vi "Build Dashboard Data.vi"(11 "Dashboard Enables":T3={"Analog Module 1"=[TRUE, TRUE, TRUE, TRUE, TRUE, TRUE, TRUE, TRUE], "Analog Module 2"=[FALSE, FALSE, FALSE, FALSE, FALSE, FALSE, FALSE, FALSE], "Digital Module 1"=TRUE, "Digital Module 2"=FALSE, "Solenoid Module"=FALSE, "Turret Gyro"=TRUE, "Robot Gyro"=TRUE, "Left Encoder"=TRUE, "Launcher Rate"=TRUE, "Right Encoder"=TRUE, "Drive Distance"=TRUE, "Selected Target"=TRUE, "Target Info"=TRUE, "Target Distance"=TRUE, "Bounding Box"=TRUE}) -> ()   [LabVIEW 2012]
doc: "This VI builds data and sends it back to the dashboard PC program. By default it sends back the raw values for the first analog, digital, and solenoid module. Modify it to send back the data you want to view. Consider adding higher level data to the Dashboard Datatype.ctl and to this VI. Then update the Dashboard to display the data however you like.\n\nThis software is licensed. Open the labview\\readme\\WPI Robotics Library Open Source License.txt file for more information."
uses:
  Dashboard Datatype.ctl
  <vilib>/Rock Robotics/WPI/DriverStation/WPI_DriverStationDigitalData.ctl
  <vilib>/Rock Robotics/SystemInterfaces/System/FPGA_SystemGet.vi
  Robot Global Data.vi
panel:
  out "Dashboard Data":T1
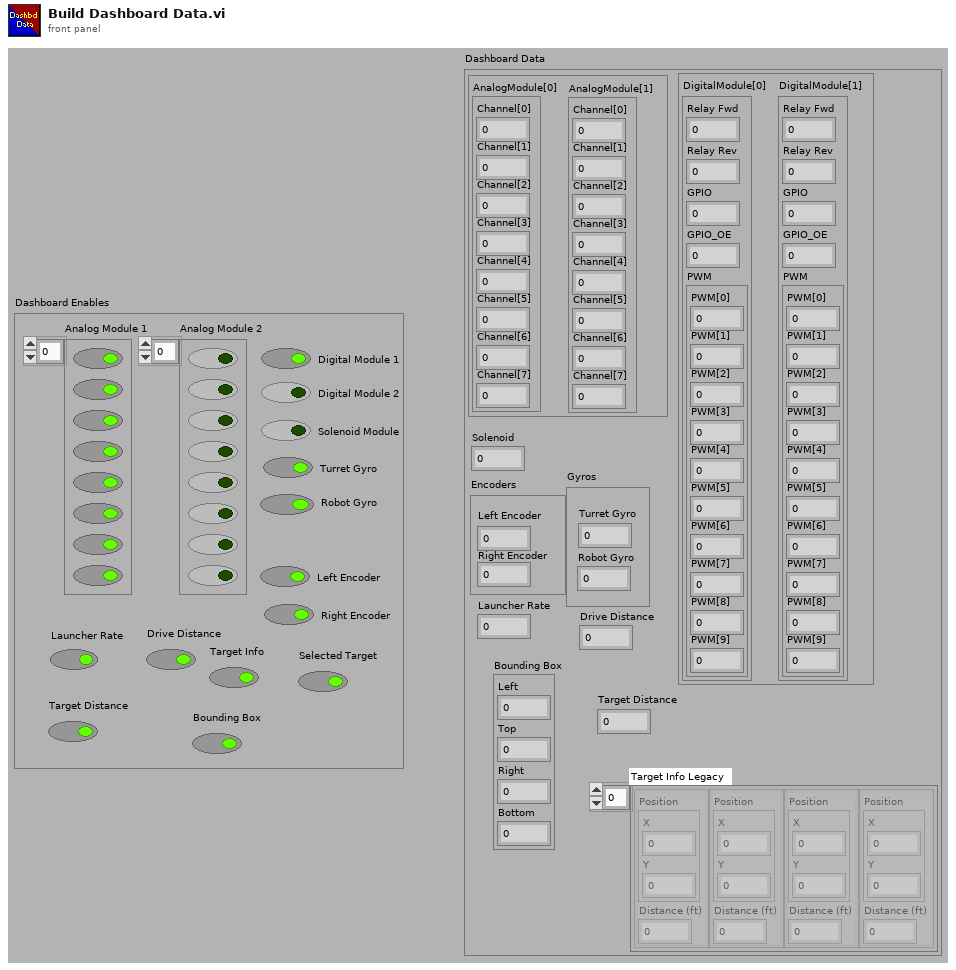
[diagram p1: front panel]
types:
  T1 = typedef "Dashboard Datatype.ctl" = cluster{cluster{"AnalogModule[0]":cluster{"Channel[0]":sgl, "Channel[1]":sgl, "Channel[2]":sgl, "Channel[3]":sgl, "Channel[4]":sgl, "Channel[5]":sgl, "Channel[6]":sgl, "Channel[7]":sgl}, "AnalogModule[1]":cluster{"Channel[0]":sgl, "Channel[1]":sgl, "Channel[2]":sgl, "Channel[3]":sgl, "Channel[4]":sgl, "Channel[5]":sgl, "Channel[6]":sgl, "Channel[7]":sgl}}, cluster{"DigitalModule[0]":T2, "DigitalModule[1]":T2}, "Solenoid":u8, "Launcher Rate":dbl, "Gyros":cluster{"Turret Gyro":dbl, "Robot Gyro":dbl}, "Encoders":cluster{"Left Encoder":dbl, "Right Encoder":dbl}, "Drive Distance":dbl, "Bounding Box":cluster{"Left":dbl, "Top":dbl, "Right":dbl, "Bottom":dbl}, "Target Distance":dbl, "Target Info Legacy":cluster{"Position":cluster{"X":dbl, "Y":dbl}, "Distance (ft)":dbl}[]}
  T2 = typedef "WPI_DriverStationDigitalData.ctl" = cluster{"Relay Fwd":u8, "Relay Rev":u8, "GPIO":u16, "GPIO_OE":u16, "PWM":cluster{"PWM[0]":u8, "PWM[1]":u8, "PWM[2]":u8, "PWM[3]":u8, "PWM[4]":u8, "PWM[5]":u8, "PWM[6]":u8, "PWM[7]":u8, "PWM[8]":u8, "PWM[9]":u8}}
  T3 = cluster{"Analog Module 1":bool[], "Analog Module 2":bool[], "Digital Module 1":bool, "Digital Module 2":bool, "Solenoid Module":bool, "Turret Gyro":bool, "Robot Gyro":bool, "Left Encoder":bool, "Launcher Rate":bool, "Right Encoder":bool, "Drive Distance":bool, "Selected Target":bool, "Target Info":bool, "Target Distance":bool, "Bounding Box":bool}
  T4 = cluster{"AnalogModule[0]":cluster{"Channel[0]":sgl, "Channel[1]":sgl, "Channel[2]":sgl, "Channel[3]":sgl, "Channel[4]":sgl, "Channel[5]":sgl, "Channel[6]":sgl, "Channel[7]":sgl}, "AnalogModule[1]":cluster{"Channel[0]":sgl, "Channel[1]":sgl, "Channel[2]":sgl, "Channel[3]":sgl, "Channel[4]":sgl, "Channel[5]":sgl, "Channel[6]":sgl, "Channel[7]":sgl}}
  T5 = cluster{"Channel[0]":sgl, "Channel[1]":sgl, "Channel[2]":sgl, "Channel[3]":sgl, "Channel[4]":sgl, "Channel[5]":sgl, "Channel[6]":sgl, "Channel[7]":sgl}[]
  T6 = cluster{"Channel[0]":sgl, "Channel[1]":sgl, "Channel[2]":sgl, "Channel[3]":sgl, "Channel[4]":sgl, "Channel[5]":sgl, "Channel[6]":sgl, "Channel[7]":sgl}
  T7 = cluster{"AnalogModule[0][0]":sgl, "AnalogModule[0][1]":sgl, "AnalogModule[0][2]":sgl, "AnalogModule[0][3]":sgl, "AnalogModule[0][4]":sgl, "AnalogModule[0][5]":sgl, "AnalogModule[0][6]":sgl, "AnalogModule[0][7]":sgl}
  T8 = cluster{"[0]":cluster{"Channel[0]":sgl, "Channel[1]":sgl, "Channel[2]":sgl, "Channel[3]":sgl, "Channel[4]":sgl, "Channel[5]":sgl, "Channel[6]":sgl, "Channel[7]":sgl}, "[1]":cluster{"Channel[0]":sgl, "Channel[1]":sgl, "Channel[2]":sgl, "Channel[3]":sgl, "Channel[4]":sgl, "Channel[5]":sgl, "Channel[6]":sgl, "Channel[7]":sgl}}
  T9 = cluster{"DigitalModule[0]":T2, "DigitalModule[1]":T2}
  T10 = typedef "FPGA_DIODevRef.ctl" = cluster{"DevStatus":errorcluster, "Module":T11}
  T11 = typedef "FPGA_TypedefDigitalModule.ctl" = enum16{"Digital Module 1", "Digital Module 2"}
  T12 = cluster{"[0]":u8, "[1]":u8, "[2]":u8, "[3]":u8, "[4]":u8, "[5]":u8, "[6]":u8, "[7]":u8, "[8]":u8, "[9]":u8}
  T13 = cluster{"Left":dbl, "Top":dbl, "Right":dbl, "Bottom":dbl}
  T14 = typedef "FPGA_SolenoidDevRef.ctl" = cluster{"DevStatus":errorcluster, "Module":T15}
  T15 = typedef "FPGA_TypedefSolenoidModule.ctl" = enum16{"Solenoid Module 1", "Solenoid Module 2"}
  T16 = cluster{"Position":cluster{"X":dbl, "Y":dbl}, "Distance (ft)":dbl}[]
  T17 = typedef "WPI_GyroDevRef.ctl" = cluster{"DevStatus":errorcluster, "Analog Module":T18, "Analog Channel":T19, "Offset":dbl, "Gain (VoltsPerDegree/Second)":dbl}
  T18 = typedef "FPGA_TypedefAnalogModule.ctl" = enum16{"Analog Module 1", "Analog Module 2"}
  T19 = typedef "FPGA_AIChannel.ctl" = enum8{"AI 1", "AI 2", "AI 3", "AI 4", "AI 5", "AI 6", "AI 7", "AI 8", "Invalid"}
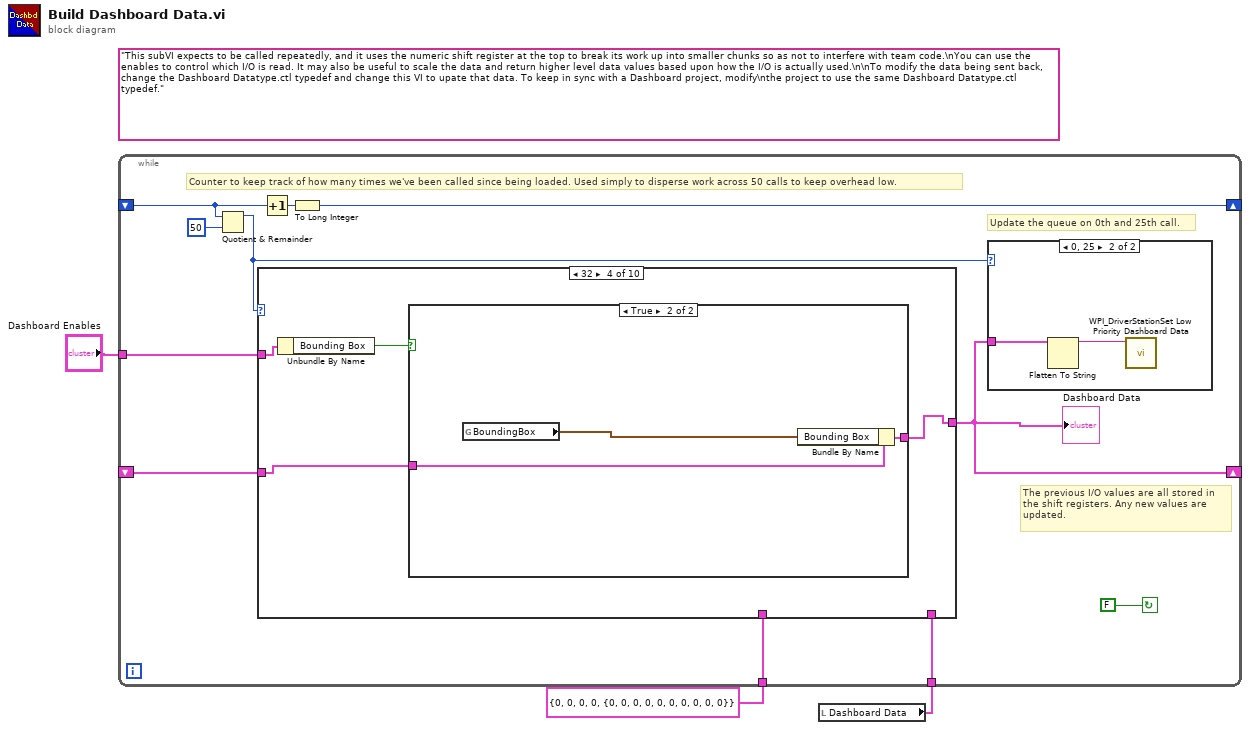
[diagram p0: block diagram]
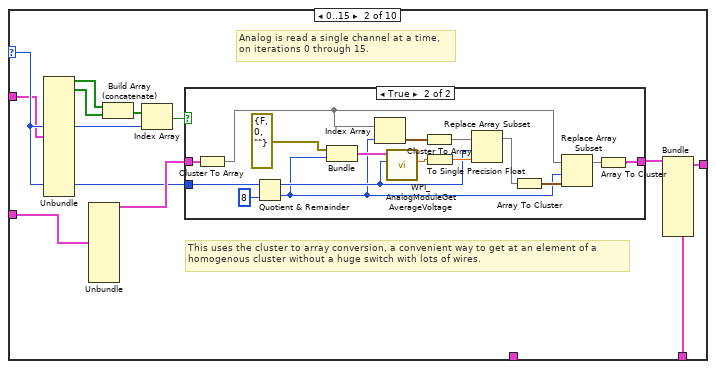
[diagram p4: hidden frame]
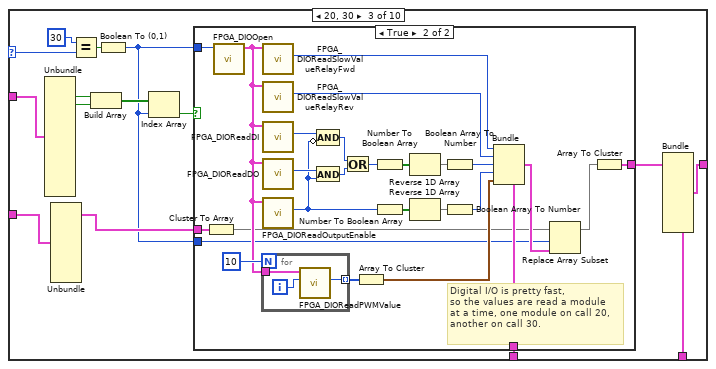
[diagram p6: hidden frame]
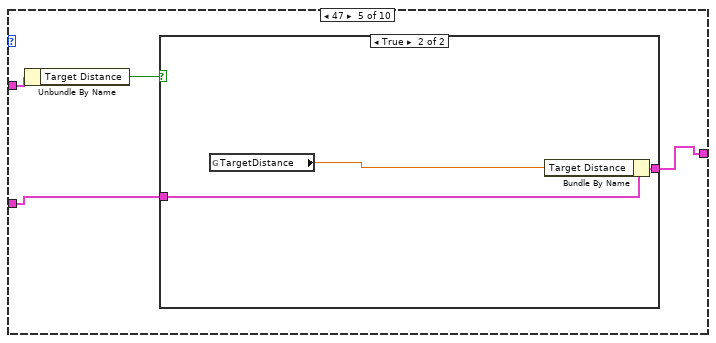
[diagram p9: hidden frame]
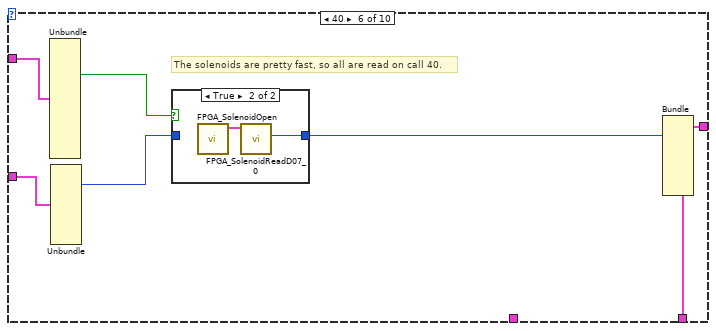
[diagram p11: hidden frame]
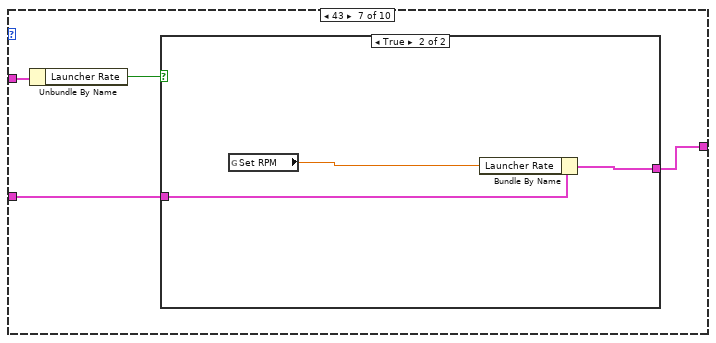
[diagram p13: hidden frame]
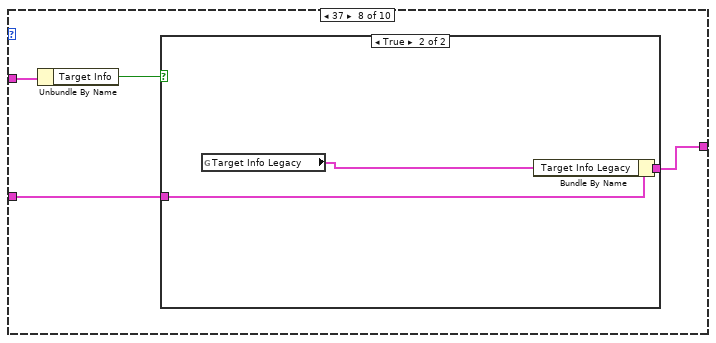
[diagram p15: hidden frame]
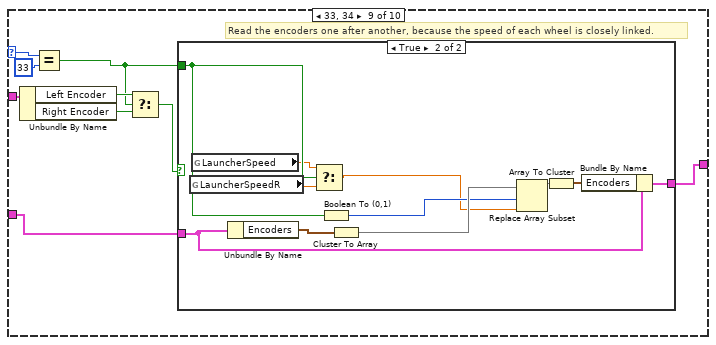
[diagram p17: hidden frame]
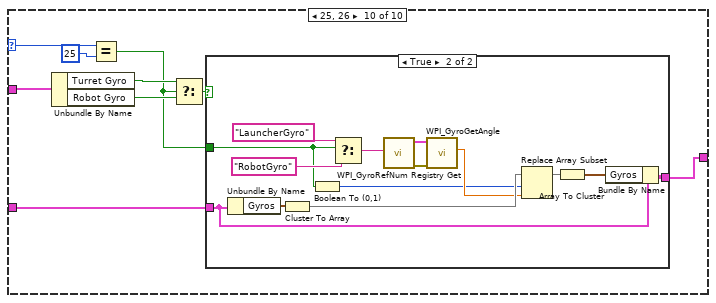
[diagram p19: hidden frame]
diagram:
  (unwired) "This subVI expects to be called repeatedly, and it uses the numeric shift register at the top to break its work up into smaller chunks so as not to interfere with team code.\nYou can use the enables to control which I/O is read. It may also be useful to scale the data and return higher level data values based upon how the I/O is actually used.\n\nTo modify the data being sent back, change the Dashboard Datatype.ctl typedef and change this VI to upate that data. To keep in sync with a Dashboard project, modify\nthe project to use the same Dashboard Datatype.ctl typedef."
  n1 = local read "Dashboard Data"() -> (w2:T1)
  n2 = while {
    shift-right: [w7] -> _
    shift-left: _ -> [w9]
    shift-right: [w4] -> _
    shift-left: _ -> [w12]
    tunnel: T2 {"Relay Fwd"=0, "Relay Rev"=0, "GPIO"=0, "GPIO_OE"=0, "PWM"={"PWM[0]"=0, "PWM[1]"=0, "PWM[2]"=0, "PWM[3]"=0, "PWM[4]"=0, "PWM[5]"=0, "PWM[6]"=0, "PWM[7]"=0, "PWM[8]"=0, "PWM[9]"=0}} ("DigitalModule[1]") -> [w11]
    tunnel: w2 -> [w6]
    tunnel: "Dashboard Enables" -> [w5]
    stop <- FALSE continue-if-true
    # "Counter to keep track of how many times we've been called since being loaded. Used simply to disperse work across 50 calls to keep overhead low."
    # "Update the queue on 0th and 25th call."
    # "The previous I/O values are all stored in\nthe shift registers. Any new values are\nupdated."
    n3 = Quotient & Remainder(x=w9, y=50) -> (x-y*floor(x/y)=w8:i32)  [unwired: 1 out]
    n4 = case shown="32" w8 {
      selector: w8 -> [_ w23 w56 _ _ _ _ _ w141 w159]
      tunnel: [w17 w19 w47 w93 w101 w110 w118 w126 w133 w154] -> w4
      tunnel: w12 -> [w17 w18 w49 w92 w100 w112 w117 w125 w134 w155]
      tunnel: w11 -> [_ _ w60 _ _ _ _ _ _ _]
      tunnel: w6 -> [_ w25 w48 _ _ w109 _ _ _ _]
      tunnel: w5 -> [_ w22 w54 w91 w99 w113 w120 w128 w139 w162]
      frame Default {
        # "Don't update any I/O"
      }
      frame 0..15 {
        # "This uses the cluster to array conversion, a convenient way to get at an element of a\nhomogenous cluster without a huge switch with lots of wires."
        # "Analog is read a single channel at a time,\non iterations 0 through 15."
        n5 = Unbundle(w22) -> ("Analog Module 1"=w21:bool[], "Analog Module 2"=w20:bool[])  [unwired: 13 out]
        n6 = Unbundle(w18) -> (w24:T4)  [unwired: 9 out]
        n7 = Build Array (concatenate)(w21, w20) -> (w27:bool[])
        n8 = Index Array(array=w27, index=w23) -> (element=w28:bool)
        n9 = case shown="True" w28 {
          tunnel: w23 -> [_ w36]
          tunnel: [w29 w33] -> w26
          tunnel: w24 -> [w29 w32]
          frame False {
          }
          frame True {
            n10 = Cluster To Array(cluster=w32) -> (array=w30:T5)
            n11 = Quotient & Remainder(x=w36, y=8) -> (x-y*floor(x/y)=w35:i32, floor(x/y)=w31:i32)
            n12 = Bundle("DevStatus"=errorcluster {"status"=FALSE, "code"=0, "source"=""}, w31) -> (w44:cluster{"DevStatus":errorcluster, i32})  [unwired: 1 out]
            n13 = Index Array(array=w30, index=w31) -> (element=w38:T6)
            n14 = call <vilib>:"WPI_AnalogModuleGetAverageVoltage.vi"("Channel"=w35, "AnalogModuleDevStatus"=w44) -> ("Average Voltage"=w41:dbl)  [unwired: 1 in, 8 out]
            n15 = Cluster To Array(cluster=w38) -> (array=w37:sgl[])
            n16 = To Single Precision Float(number=w41) -> (single precision float=w40:sgl)
            n17 = Replace Array Subset(array=w37, new element=w40, index=w35) -> (w39:sgl[])
            n18 = Array To Cluster(array=w39) -> (cluster=w43:T7)
            n19 = Replace Array Subset(array=w30, new element=w43, index=w31) -> (w34:T5)
            n20 = Array To Cluster(array=w34) -> (cluster=w33:T8)
          }
        }
        n21 = Bundle(cluster=w25, w26) -> (w19:T1)  [unwired: 9 out]
      }
      frame 20, 30 {
        n22 = Unbundle(w54) -> ("Digital Module 1"=w53:bool, "Digital Module 2"=w52:bool)  [unwired: 13 out]
        n23 = Unbundle(w49) -> (w51:T9)  [unwired: 9 out]
        n24 = Equal?(x=30, y=w56) -> (x = y?=w58:bool)
        n25 = Build Array(w53, w52) -> (w55:bool[])
        n26 = Boolean To (0,1)(Boolean=w58) -> (0, 1=w46:i16)
        n27 = Index Array(array=w55, index=w46) -> (element=w57:bool)
        n28 = case shown="True" w57 {
          tunnel: w60 -> [_ w69]
          tunnel: [w61 w62] -> w50
          tunnel: w46 -> [_ w67]
          tunnel: w46 -> [_ w66]
          tunnel: w51 -> [w61 w65]
          frame False {
          }
          frame True {
            # "Digital I/O is pretty fast,\nso the values are read a module\nat a time, one module on call 20,\nanother on call 30."
            n29 = Cluster To Array(cluster=w65) -> (array=w64:T2[])
            n30 = call <vilib>:"FPGA_DIOOpen.vi"("Module (Module 1)"=w67) -> ("DIODeviceRef"=w85:T10)  [unwired: 1 in, 9 out]
            n31 = for {
              N: 10 -> [_]
              tunnel: w85 -> [w90]
              tunnel: [w88] -> w86 mode=indexing
              i -> [w89]
              n32 = call <vilib>:"FPGA_DIOReadPWMValue.vi"("PWMChannel"=w89, "DIODeviceRef In"=w90) -> ("PWMValue"=w88:u8)  [unwired: 1 in, 8 out]
            }
            n33 = call <vilib>:"FPGA_DIOReadSlowValueRelayFwd.vi"("DIODeviceRef In"=w85) -> ("Relay Forward"=w78:u8)  [unwired: 1 in, 9 out]
            n34 = call <vilib>:"FPGA_DIOReadSlowValueRelayRev.vi"("DIODeviceRef In"=w85) -> ("Relay Reverse"=w79:u8)  [unwired: 1 in, 9 out]
            n35 = call <vilib>:"FPGA_DIOReadDI.vi"("DIODeviceRef In"=w85) -> ("DI"=w83:u16)  [unwired: 1 in, 9 out]
            n36 = call <vilib>:"FPGA_DIOReadDO.vi"("DIODeviceRef In"=w85) -> ("DO"=w82:u16)  [unwired: 1 in, 9 out]
            n37 = call <vilib>:"FPGA_DIOReadOutputEnable.vi"("DIODeviceRef In"=w85) -> ("OutputEnable"=w73:u16)  [unwired: 1 in, 9 out]
            n38 = And(x=w82, y=w73) -> (x .and. y?=w81:u16)
            n39 = Compound Arithmetic op=AND(w83, invert w73) -> (w80:u16)
            n40 = Or(x=w80, y=w81) -> (x .or. y?=w71:u16)
            n41 = Array To Cluster(array=w86) -> (cluster=w84:T12)
            n42 = Number To Boolean Array(number=w71) -> (Boolean array=w76:bool[])
            n43 = Number To Boolean Array(number=w73) -> (Boolean array=w75:bool[])
            n44 = Reverse 1D Array(array=w76) -> (reversed array=w77:bool[])
            n45 = Reverse 1D Array(array=w75) -> (reversed array=w74:bool[])
            n46 = Boolean Array To Number(Boolean array=w77) -> (number=w70:u32)
            n47 = Boolean Array To Number(Boolean array=w74) -> (number=w72:u32)
            n48 = Bundle(cluster=w69, "Relay Fwd"=w78, "Relay Rev"=w79, "GPIO"=w70, "GPIO_OE"=w72, "PWM"=w84) -> (w68:T2)
            n49 = Replace Array Subset(array=w64, new element=w68, index=w66) -> (w63:T2[])
            n50 = Array To Cluster(array=w63) -> (cluster=w62:cluster{"[0]":T2, "[1]":T2})
          }
        }
        n51 = Bundle(cluster=w48, w50) -> (w47:T1)  [unwired: 9 out]
      }
      frame 32 {
        n52 = Unbundle By Name(w91) -> ("Bounding Box"=w94:bool)
        n53 = case shown="True" w94 {
          tunnel: [w95 w98] -> w93
          tunnel: w92 -> [w95 w97]
          frame False {
          }
          frame True {
            n54 = global read "Robot Global Data.vi" "BoundingBox"() -> (w96:T13)
            n55 = Bundle By Name(cluster=w97, "Bounding Box"=w96) -> (w98:T1)
          }
        }
      }
      frame 47 {
        n56 = Unbundle By Name(w99) -> ("Target Distance"=w102:bool)
        n57 = case shown="True" w102 {
          tunnel: [w103 w106] -> w101
          tunnel: w100 -> [w103 w105]
          frame False {
          }
          frame True {
            n58 = global read "Robot Global Data.vi" "TargetDistance"() -> (w104:dbl)
            n59 = Bundle By Name(cluster=w105, "Target Distance"=w104) -> (w106:T1)
          }
        }
      }
      frame 40 {
        # "The solenoids are pretty fast, so all are read on call 40."
        n60 = Unbundle(w113) -> ("Solenoid Module"=w107:bool)  [unwired: 14 out]
        n61 = Unbundle(w112) -> ("Solenoid"=w111:u8)  [unwired: 9 out]
        n62 = case shown="True" w107 {
          tunnel: [w114 w115] -> w108
          tunnel: w111 -> [w114 _]
          frame False {
          }
          frame True {
            n63 = call <vilib>:"FPGA_SolenoidOpen.vi"() -> ("SolenoidDevRef"=w116:T14)  [unwired: 2 in, 9 out]
            n64 = call <vilib>:"FPGA_SolenoidReadD07_0.vi"("SolenoidDevRef"=w116) -> ("DO7:0"=w115:u8)  [unwired: 1 in, 9 out]
          }
        }
        n65 = Bundle(cluster=w109, "Solenoid"=w108) -> (w110:T1)  [unwired: 9 out]
      }
      frame 43 {
        n66 = Unbundle By Name(w120) -> ("Launcher Rate"=w119:bool)
        n67 = case shown="True" w119 {
          tunnel: [w121 w124] -> w118
          tunnel: w117 -> [w121 w123]
          frame False {
          }
          frame True {
            n68 = global read "Robot Global Data.vi" "Set RPM"() -> (w122:dbl)
            n69 = Bundle By Name(cluster=w123, "Launcher Rate"=w122) -> (w124:T1)
          }
        }
      }
      frame 37 {
        n70 = Unbundle By Name(w128) -> ("Target Info"=w127:bool)
        n71 = case shown="True" w127 {
          tunnel: [w129 w132] -> w126
          tunnel: w125 -> [w129 w131]
          frame False {
          }
          frame True {
            n72 = global read "Robot Global Data.vi" "Target Info Legacy"() -> (w130:T16)
            n73 = Bundle By Name(cluster=w131, "Target Info Legacy"=w130) -> (w132:T1)
          }
        }
      }
      frame 33, 34 {
        # "Read the encoders one after another, because the speed of each wheel is closely linked."
        n74 = Unbundle By Name(w139) -> ("Left Encoder"=w137:bool, "Right Encoder"=w138:bool)
        n75 = Equal?(x=w141, y=33) -> (x = y?=w136:bool)
        n76 = Select(t=w137, s=w136, f=w138) -> (s? t:f=w135:bool)
        n77 = case shown="True" w135 {
          tunnel: w136 -> [_ w151]
          tunnel: w134 -> [w142 w148]
          tunnel: [w142 w147] -> w133
          frame False {
          }
          frame True {
            n78 = global read "Robot Global Data.vi" "LauncherSpeedR"() -> (w145:dbl)
            n79 = global read "Robot Global Data.vi" "LauncherSpeed"() -> (w144:dbl)
            n80 = Unbundle By Name(w148) -> ("Encoders"=w153:cluster{"Left Encoder":dbl, "Right Encoder":dbl})
            n81 = Select(t=w144, s=w151, f=w145) -> (s? t:f=w143:dbl)
            n82 = Boolean To (0,1)(Boolean=w151) -> (0, 1=w150:i16)
            n83 = Cluster To Array(cluster=w153) -> (array=w152:dbl[])
            n84 = Replace Array Subset(array=w152, new element=w143, index=w150) -> (w149:dbl[])
            n85 = Array To Cluster(array=w149) -> (cluster=w146:cluster{"Encoders[0]":dbl, "Encoders[1]":dbl})
            n86 = Bundle By Name(cluster=w148, "Encoders"=w146) -> (w147:T1)
          }
        }
      }
      frame 25, 26 {
        n87 = Unbundle By Name(w162) -> ("Turret Gyro"=w161:bool, "Robot Gyro"=w160:bool)
        n88 = Equal?(x=w159, y=25) -> (x = y?=w156:bool)
        n89 = Select(t=w161, s=w156, f=w160) -> (s? t:f=w157:bool)
        n90 = case shown="True" w157 {
          tunnel: w156 -> [_ w172]
          tunnel: w155 -> [w163 w166]
          tunnel: [w163 w168] -> w154
          frame False {
          }
          frame True {
            n91 = Unbundle By Name(w166) -> ("Gyros"=w165:cluster{"Turret Gyro":dbl, "Robot Gyro":dbl})
            n92 = Cluster To Array(cluster=w165) -> (array=w171:dbl[])
            n93 = Boolean To (0,1)(Boolean=w172) -> (0, 1=w167:i16)
            n94 = Select(t="LauncherGyro", s=w172, f="RobotGyro") -> (s? t:f=w173:string)
            n95 = call <vilib>:"WPI_GyroRefNum Registry Get.vi"("refnum name"=w173) -> ("error out"=w177:errorcluster, "GyroDevRef"=w176:T17)  [unwired: 9 in]
            n96 = call <vilib>:"WPI_GyroGetAngle.vi"("error in (no error)"=w177, "GyroDevRef"=w176) -> ("Angle"=w170:dbl)  [unwired: 6 in, 3 out]
            n97 = Replace Array Subset(array=w171, new element=w170, index=w167) -> (w169:dbl[])
            n98 = Array To Cluster(array=w169) -> (cluster=w164:cluster{"Gyros[0]":dbl, "Gyros[1]":dbl})
            n99 = Bundle By Name(cluster=w166, "Gyros"=w164) -> (w168:T1)
          }
        }
      }
    }
    "Dashboard Data" <- w4
    n100 = Increment(x=w9) -> (x+1=w14:i32)
    n101 = To Long Integer(number=w14) -> (32bit integer=w7:i32)
    n102 = case shown="0, 25" w8 {
      tunnel: w4 -> [_ w16]
      frame Default {
      }
      frame 0, 25 {
        n103 = Flatten To String(anything=w16) -> (data string=w15:string)  [unwired: 1 in, 4 out]
        n104 = call <vilib>:"WPI_DriverStationSet Low Priority Dashboard Data.vi"("User Data"=w15) -> ()  [unwired: 1 in, 10 out]
      }
    }
  }
